vi "MEASRSLT.vi"(0 "VISA resource name":refnum<visa-resource-name>, 1 "Measurement Type":string(combo)="FREQ - frequency (Hz)", 7 "error in (no error)":errorcluster) -> (20 "VISA resource name out":refnum<visa-resource-name>, 21 "Measurement Result":string="\r\n", 22 "Measurement Result":dbl caption="FREQ Measurement Result (Hz)", 23 "Unit":string, 25 "Error Message":string, 26 "Error Code":i32, 27 "error out":errorcluster)   [LabVIEW 2010, in "VITREK V7X.lvlib"]
doc: "Responds with a <NR3> measurement reslut during execution of a a test step. <STRING> is -\nFREQ - frequency (in Hz)\nAMPS - DC or RMS current (in Amps)\nVOLTS - DC or RMS voltage (in Volts)\nOHMS - DC or RMS impedance (in ohms)\nARC - highest ARC current (in Amps).\n\n<b>Note:</b> please refer to the instrument manual for the <b>MEASRSLT?,<STRING></b> specification."
uses:
  VITREK V7X.lvlib
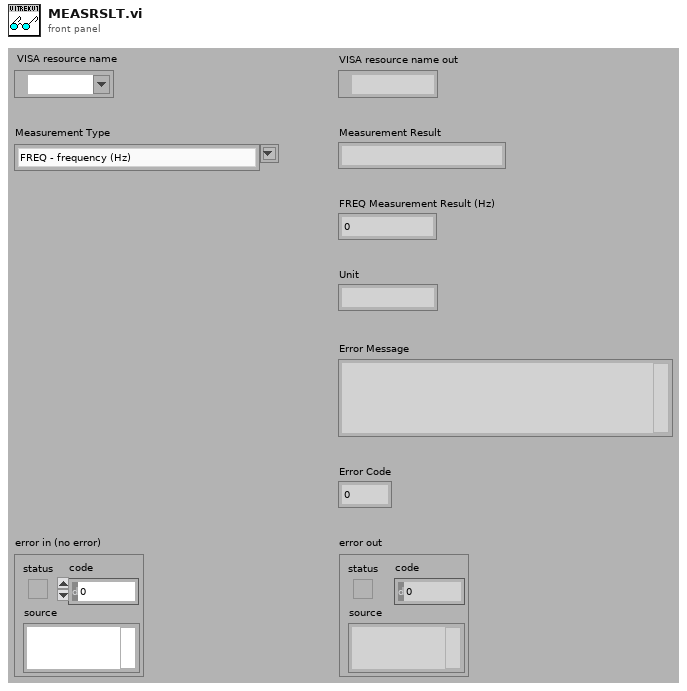
[diagram p1: front panel]
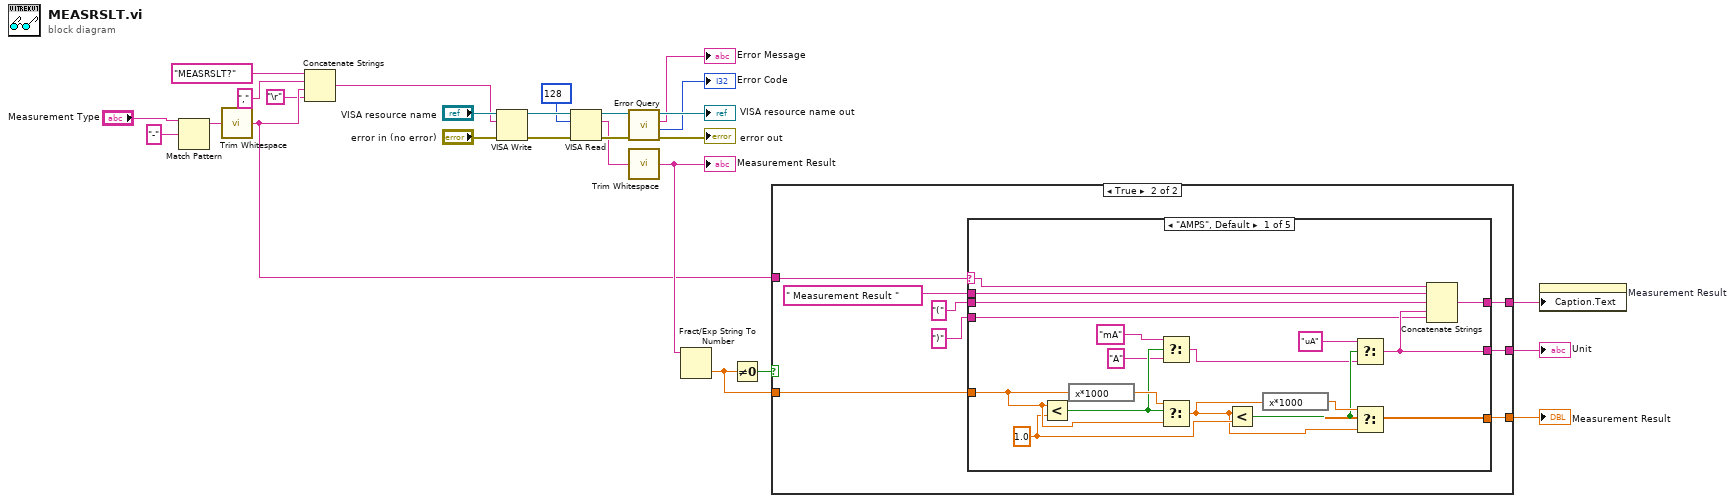
[diagram p0: block diagram]
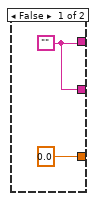
[diagram p2: hidden frame]
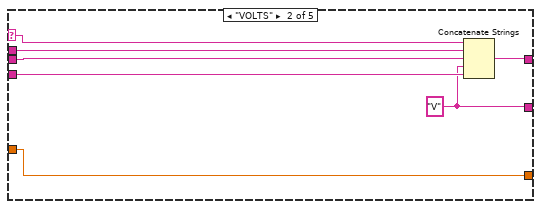
[diagram p3: hidden frame]
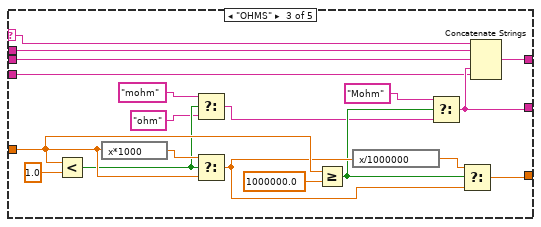
[diagram p4: hidden frame]
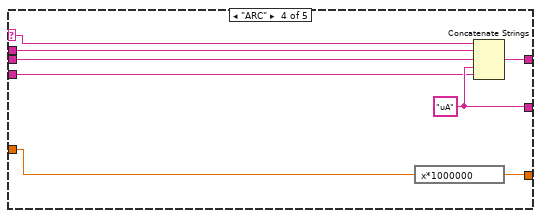
[diagram p5: hidden frame]
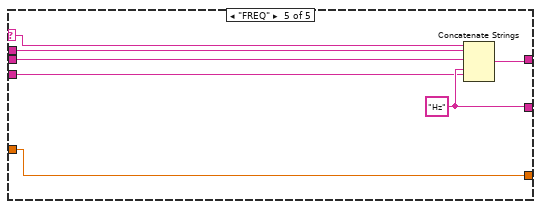
[diagram p6: hidden frame]
diagram:
  n1 = Match Pattern(string="Measurement Type", regular expression="-") -> (before substring=w11:string)  [unwired: 1 in, 3 out]
  n2 = call <vilib>:"Trim Whitespace.vi"("string"=w11) -> ("trimmed string"=w9:string)  [unwired: 1 in]
  n3 = Concatenate Strings("MEASRSLT?", ",", w9, "\r") -> (w16:string)
  n4 = VISA Write(VISA resource name="VISA resource name", write buffer=w16, error in (no error)="error in (no error)") -> (VISA resource name out=w22:refnum<visa-resource-name>, error out=w20:errorcluster)  [unwired: 1 out]
  n5 = VISA Read(VISA resource name=w22, byte count=u32 128, error in (no error)=w20) -> (VISA resource name out=w21:refnum<visa-resource-name>, read buffer=w17:string, error out=w18:errorcluster)  [unwired: 1 out]
  n6 = call "Error Query.vi"("error in (no error)"=w18, "VISA resource name"=w21) -> ("error out"=→"error out":errorcluster, "Error Code"=→"Error Code":i32, "Error Message"=→"Error Message":string, "VISA resource name out"=→"VISA resource name out":refnum<visa-resource-name>)  [unwired: 6 in]
  n7 = call <vilib>:"Trim Whitespace.vi"("string"=w17) -> ("trimmed string"=w10:string)  [unwired: 1 in]
  "Measurement Result" <- w10
  n8 = Fract/Exp String To Number(string=w10) -> (number=w5:dbl)  [unwired: 3 in, 1 out]
  n9 = Not Equal To 0?(x=w5) -> (x != 0?=w4:bool)
  n10 = case shown="True" w4 {
    tunnel: w9 -> [_ w36]
    tunnel: [0.0 w35] -> w8
    tunnel: [w27 w34] -> w7
    tunnel: [w27 w33] -> w6
    tunnel: w5 -> [_ w29]
    frame False {
      w27 = ""
    }
    frame True {
      n11 = case shown="\"AMPS\", Default" w36 {
        selector: w36 -> [w48 w60 w63 w85 w93]
        tunnel: w29 -> [w54 w61 w76 w87 w95]
        tunnel: [w49 w61 w78 w88 w95] -> w35
        tunnel: [w41 w59 w66 w86 w94] -> w34
        tunnel: [w40 w56 w67 w84 w92] -> w33
        tunnel: "(" -> [w39 w58 w64 w81 w91]
        tunnel: ")" -> [w38 w57 w65 w83 w90]
        tunnel: " Measurement Result " -> [w37 w55 w62 w82 w89]
        frame "AMPS", Default {
          w52 = 1.0 ("y")
          n12 = Less?(x=w54, y=w52) -> (x < y?=w46:bool)
          n13 = expression code="x*1000"(w54) -> (w50:dbl)
          n14 = Select(t="mA", s=w46, f="A") -> (s? t:f=w42:string)
          n15 = Select(t=w50, s=w46, f=w54) -> (s? t:f=w51:dbl)
          n16 = Less?(x=w51, y=w52) -> (x < y?=w44:bool)
          n17 = expression code="x*1000"(w51) -> (w53:dbl)
          n18 = Select(t="uA", s=w44, f=w42) -> (s? t:f=w40:string)
          n19 = Select(t=w53, s=w44, f=w51) -> (s? t:f=w49:dbl)
          n20 = Concatenate Strings(w48, w37, w39, w40, w38) -> (w41:string)
        }
        frame "VOLTS" {
          w56 = "V"
          n21 = Concatenate Strings(w60, w55, w58, w56, w57) -> (w59:string)
        }
        frame "OHMS" {
          n22 = Less?(x=w76, y=1.0) -> (x < y?=w73:bool)
          n23 = expression code="x*1000"(w76) -> (w77:dbl)
          n24 = Select(t="mohm", s=w73, f="ohm") -> (s? t:f=w68:string)
          n25 = Select(t=w77, s=w73, f=w76) -> (s? t:f=w74:dbl)
          n26 = Greater Or Equal?(x=w76, y=1000000.0) -> (x >= y?=w70:bool)
          n27 = expression code="x/1000000"(w74) -> (w75:dbl)
          n28 = Select(t="Mohm", s=w70, f=w68) -> (s? t:f=w67:string)
          n29 = Select(t=w75, s=w70, f=w74) -> (s? t:f=w78:dbl)
          n30 = Concatenate Strings(w63, w62, w64, w67, w65) -> (w66:string)
        }
        frame "ARC" {
          w84 = "uA"
          n31 = expression code="x*1000000"(w87) -> (w88:dbl)
          n32 = Concatenate Strings(w85, w82, w81, w84, w83) -> (w86:string)
        }
        frame "FREQ" {
          w92 = "Hz"
          n33 = Concatenate Strings(w93, w89, w91, w92, w90) -> (w94:string)
        }
      }
    }
  }
  "Measurement Result" <- w8
  "Unit" <- w6
  n34 = property on="Measurement Result" class="DigNum (strict)"("Caption.Text"=w7) -> ()  [unwired: 2 in, 2 out]
